vi "Gauss Function.vi"(4 "c":dbl format="%.2f", 5 "b":dbl format="%.2f", 6 "a":dbl format="%.2f", 7 "x":dbl format="%.2f") -> (3 "F(x, a, b, c)":dbl format="%.2f")   [LabVIEW 2017, in "NI_Gmath.lvlib"]
doc: "Computes the Gauss hypergeometric function <B>F(x, a, b, c)</B> according to the input argument and parameters you specify."
uses:
  NI_Gmath.lvlib
  lvanlys.dll
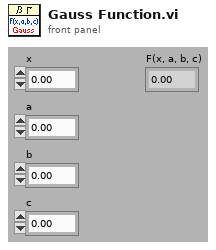
[diagram p1: front panel]
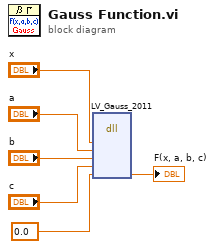
[diagram p0: block diagram]
diagram:
  n1 = dll-call lib="C:/Program Files/National Instruments/LabVIEW 2017/resource/lvanlys.*" fn="LV_Gauss_2011"("x"="x", "a"="a", "b"="b", "c"="c", "Gauss(x, a, b, c)"=0.0 ("Gauss")) -> ("Gauss(x, a, b, c)"=→"F(x, a, b, c)":dbl)  [unwired: 8 in, 2 out]
